vi "PXI-Make Ramp.vi"(0 "Ramping":T1={"Ramp up?"=FALSE, "Ramp down?"=FALSE, "Ramp duration (msecs)"=0.0, "Ramp type"=enum."Cos2"}, 7 "Sampling rate (Hz)":dbl, 9 "# samples":u32) -> (4 "Ramping?":bool, 8 "Ramp out":dbl[](array[numeric]))   [LabVIEW 2020]
uses:
  Type Defs/Ramping Params.ctl
  <vilib>/Analysis/1siggen.llb/Ramp Pattern by Samples.vi
  <vilib>/Analysis/NI_AALBase.lvlib
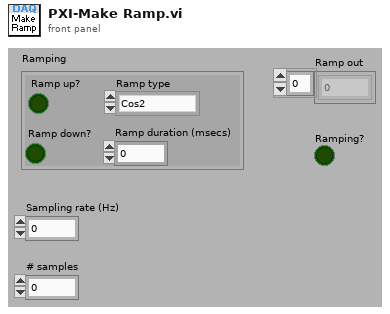
[diagram p1: front panel]
types:
  T1 = typedef "Ramping Params.ctl" = cluster{"Ramp up?":bool, "Ramp down?":bool, "Ramp duration (msecs)":dbl, "Ramp type":enum16{"Linear", "Cos2"}}
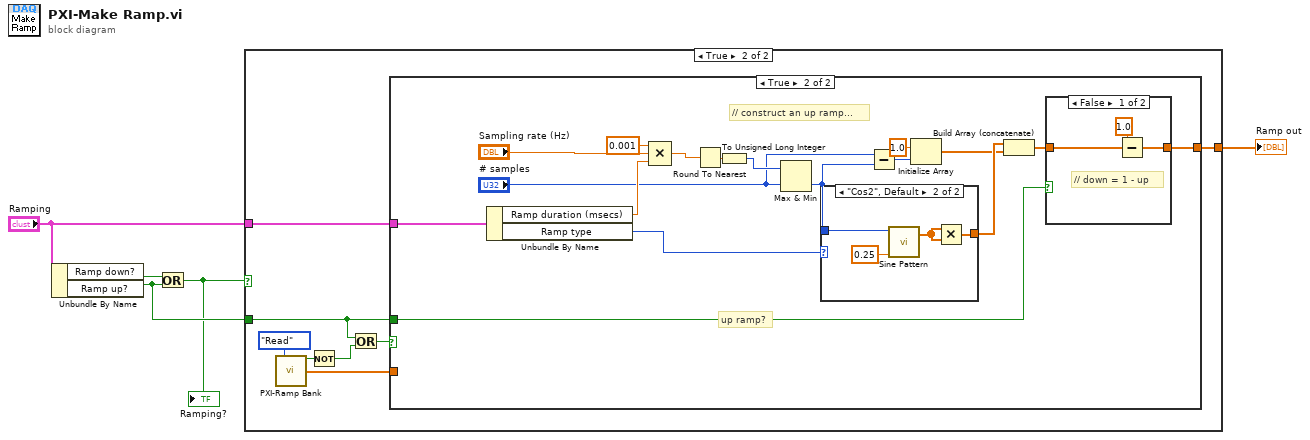
[diagram p0: block diagram]
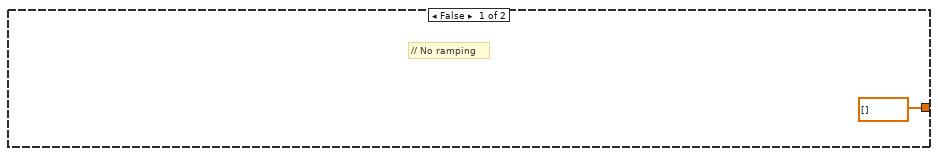
[diagram p2: hidden frame]
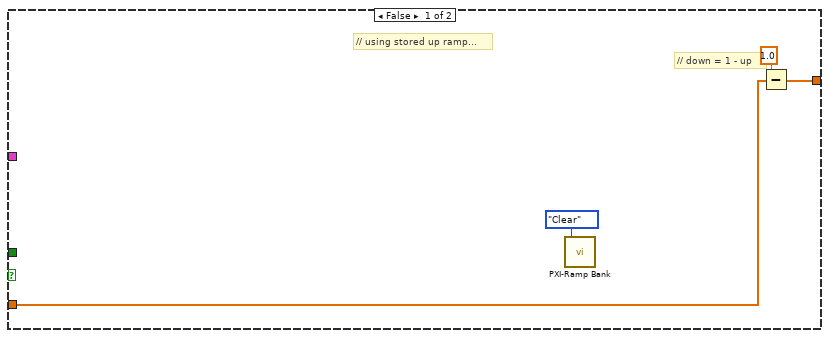
[diagram p3: hidden frame]
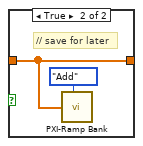
[diagram p4: hidden frame]
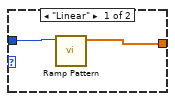
[diagram p5: hidden frame]
diagram:
  n1 = Unbundle By Name("Ramping") -> ("Ramp down?"=w5:bool, "Ramp up?"=w3:bool)
  n2 = Or(x=w5, y=w3) -> (x .or. y?=w2:bool)
  "Ramping?" <- w2
  n3 = case shown="True" w2 {
    tunnel: [dbl[] [] w9] -> w1
    tunnel: "Ramping" -> [_ w8]
    tunnel: w3 -> [_ w7]
    frame False {
      # "// No ramping"
    }
    frame True {
      n4 = call "PXI-Ramp Bank.vi"("Action"=enum16{"Add", "Read", "Clear"}."Read") -> ("Ramp available?"=w13:bool, "Ramp Out"=w10:dbl[])  [unwired: 13 in]
      n5 = Not(x=w13) -> (.not. x?=w14:bool)
      n6 = Or(x=w7, y=w14) -> (x .or. y?=w11:bool)
      n7 = case shown="True" w11 {
        tunnel: [w16 w25] -> w9
        tunnel: w10 -> [w17 _]
        tunnel: w7 -> [_ w24]
        tunnel: w8 -> [_ w20]
        frame False {
          # "// using stored up ramp..."
          # "// down = 1 - up"
          n8 = call "PXI-Ramp Bank.vi"("Action"=enum16{"Add", "Read", "Clear"}."Clear") -> ()  [unwired: 13 in, 2 out]
          n9 = Subtract(x=1.0, y=w17) -> (x-y=w16:dbl[])
        }
        frame True {
          # "up ramp?"
          # "// construct an up ramp..."
          n10 = Unbundle By Name(w20) -> ("Ramp duration (msecs)"=w35:dbl, "Ramp type"=w34:enum16{"Linear", "Cos2"})
          n11 = Compound Arithmetic op=MULTIPLY(0.001 ("value"), "Sampling rate (Hz)", w35) -> (w23:dbl)
          n12 = Round To Nearest(number=w23) -> (nearest integer value=w33:dbl)
          n13 = To Unsigned Long Integer(number=w33) -> (unsigned 32bit integer=w32:u32)
          n14 = Max & Min(x=w32, y="# samples") -> (min(x,y)=w30:u32)  [unwired: 1 out]
          n15 = case shown="\"Cos2\", Default" w34 {
            tunnel: w30 -> [w42 w46]
            tunnel: [w41 w43] -> w31
            frame "Linear" {
              n16 = call-poly <vilib>:"Ramp Pattern.vi"("samples"=w42) -> ("Ramp Pattern"=w41:dbl[])  [unwired: 9 in, 1 out]
            }
            frame "Cos2", Default {
              n17 = call <vilib>:"Sine Pattern.vi"("cycles"=0.25, "samples"=w46) -> ("Sinusoidal Pattern"=w44:dbl[])  [unwired: 2 in, 1 out]
              n18 = Multiply(x=w44, y=w44) -> (x*y=w43:dbl[])
            }
          }
          n19 = Subtract(x="# samples", y=w30) -> (x-y=w29:u32)
          n20 = Initialize Array(1.0 ("element"), w29) -> (w27:dbl[])
          n21 = Build Array (concatenate)(w31, w27) -> (w26:dbl[])
          n22 = case shown="False" w24 {
            tunnel: w26 -> [w37 w39]
            tunnel: [w36 w39] -> w25
            frame False {
              # "// down = 1 - up"
              n23 = Subtract(x=1.0, y=w37) -> (x-y=w36:dbl[])
            }
            frame True {
              # "// save for later"
              n24 = call "PXI-Ramp Bank.vi"("Action"=enum16{"Add", "Read", "Clear"}."Add", "Ramp In"=w39) -> ()  [unwired: 12 in, 2 out]
            }
          }
        }
      }
    }
  }
  "Ramp out" <- w1
